vi "checkBeginDeadBallPlayVSS.vi"(8 "error in (no error)":errorcluster, 9 "last command_interpreted":T1, 10 "Game":refnum<class "Game.lvclass">, 11 "DeadBallPlayVSS in":refnum<class "DeadBallPlayVSS.lvclass">) -> (0 "error out":errorcluster, 2 "Boolean":bool, 3 "DeadBallPlayVSS out":refnum<class "DeadBallPlayVSS.lvclass">)   [LabVIEW 2023, in "DeadBallPlayVSS.lvclass"]
uses:
  DeadBallPlayVSS.lvclass
  Game_class/Game.lvclass
  Referee_class/command_interpreted.ctl
  Utilities_class/Utilities.lvclass
  Game_class/Game.lvclass/Game.ctl
  Referee_class/Referee.lvclass/Referee.ctl
  Ball_class/Ball.lvclass/Ball.ctl
  Game_class/Read Referee.vi
  Game_class/Read BallRef.vi
  Ball_class/Read v_x.vi
  Ball_class/Read v_y.vi
  Referee_class/Read command_interpreted.vi
  Referee_class/Referee.lvclass
  Ball_class/Ball.lvclass
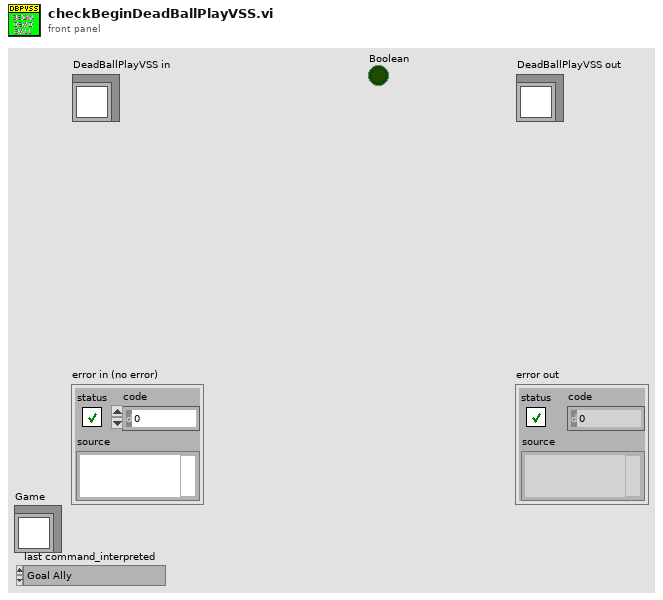
[diagram p1: front panel]
types:
  T1 = typedef "command_interpreted.ctl" = enum16{"Goal Ally", "Goal Enemy", "Ball Placement Enemy", "Ball Placement Ally", "Normal Half Time", "Extra Time  Break", "Extra Half Time", "None", "Post Game", "PKA Normal Start", "Prepare Kickoff Ally", "PKE Normal Start", "Prepare Kickoff Enemy", "Force Start", "Halt", "Timeout", "Prepare Penalty Ally", "Prepare Penalty Enemy", "PPA NormalStart", "PPE Normal Start", "Indirect Free Ally", "Direct Free Enemy", "Direct Free Ally", "Indirect Free Enemy", "Stop"}
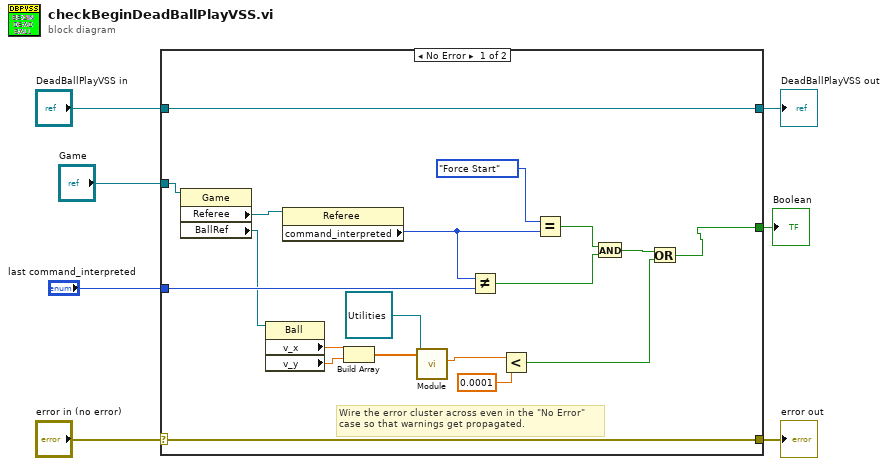
[diagram p0: block diagram]
diagram:
  n1 = case shown="No Error" "error in (no error)" {
    selector: "error in (no error)" -> [w25 w28]
    tunnel: [w25 w28] -> w6
    tunnel: [w26 w27] -> w4
    tunnel: "DeadBallPlayVSS in" -> [w26 w27]
    tunnel: "Game" -> [w18 _]
    tunnel: "last command_interpreted" -> [w19 _]
    tunnel: [w8 _] -> w1
    frame No Error {
      # "Wire the error cluster across even in the \"No Error\"\ncase so that warnings get propagated."
      n2 = property class="Game"(reference=w18) -> ("Referee"=w24:refnum<class "Referee.lvclass">, "BallRef"=w17:refnum<class "Ball.lvclass">)  [unwired: 1 in, 2 out]
      n3 = property class="Ball"(reference=w17) -> ("v_x"=w16:dbl, "v_y"=w15:dbl)  [unwired: 1 in, 2 out]
      n4 = property class="Referee"(reference=w24) -> ("command_interpreted"=w22:T1)  [unwired: 1 in, 2 out]
      n5 = Build Array(w16, w15) -> (w14:dbl[])
      n6 = call-dynamic "Module.vi"("2D vector"=w14, "Utilities in"=refnum<class "Utilities.lvclass"> refnum) -> ("Modulo"=w11:dbl)  [unwired: 7 in, 2 out]
      n7 = Not Equal?(x=w22, y=w19) -> (x != y?=w20:bool)
      n8 = Less?(x=w11, y=0.0001) -> (x < y?=w9:bool)
      n9 = Equal?(x=command_interpreted."Force Start" ("command_interpreted"), y=w22) -> (x = y?=w21:bool)
      n10 = And(x=w21, y=w20) -> (x .and. y?=w12:bool)
      n11 = Or(x=w12, y=w9) -> (x .or. y?=w8:bool)
    }
    frame Error {
    }
  }
  "error out" <- w6
  "DeadBallPlayVSS out" <- w4
  "Boolean" <- w1
